vi "stop.vi"(8 "error in (no error)":errorcluster, 11 "WriteSignalsGenericPlugin in":refnum<class "GenericSignalWriter.lvclass">) -> (0 "error out":errorcluster, 3 "WriteSignalsGenericPlugin out":refnum<class "GenericSignalWriter.lvclass">)   [LabVIEW 2010, in "GenericSignalWriter.lvclass"]
uses:
  GenericSignalWriter.lvclass
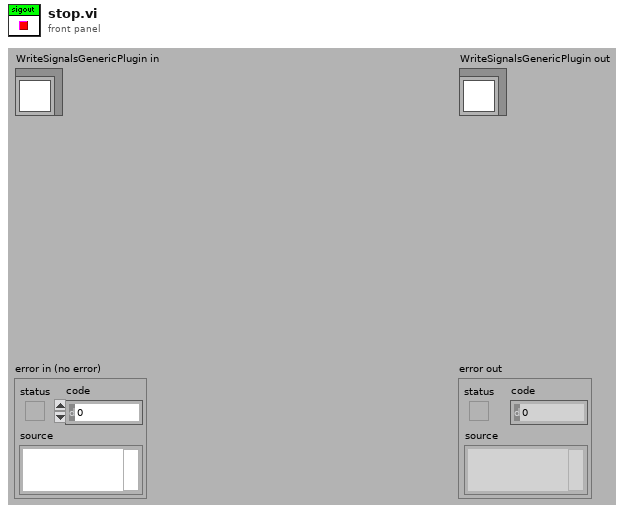
[diagram p1: front panel]
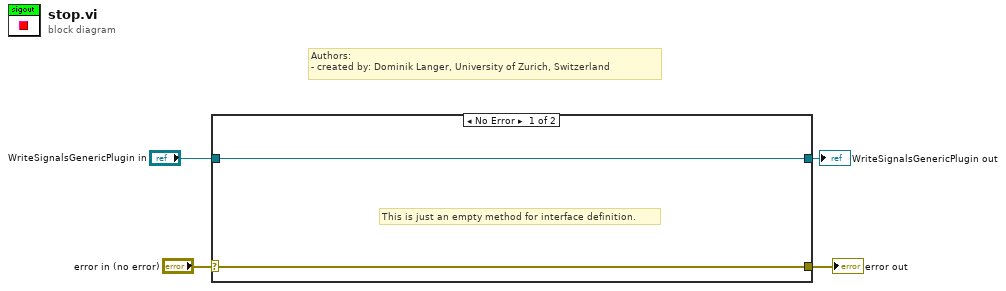
[diagram p0: block diagram]
diagram:
  # "Authors: \n- created by: Dominik Langer, University of Zurich, Switzerland"
  n1 = case shown="No Error" "error in (no error)" {
    selector: "error in (no error)" -> [w5 w8]
    tunnel: [w5 w8] -> w3
    tunnel: [w6 w7] -> w1
    tunnel: "WriteSignalsGenericPlugin in" -> [w6 w7]
    frame No Error {
      # "This is just an empty method for interface definition."
    }
    frame Error {
    }
  }
  "error out" <- w3
  "WriteSignalsGenericPlugin out" <- w1
